vi "Write plots.vi"(5 "plots":refnum<class "Plot.lvclass">[](array[class]), 9 "WaveformChart in":refnum<class "WaveformChart.lvclass">) -> (3 "WaveformChart out":refnum<class "WaveformChart.lvclass">)   [LabVIEW 2014, in "WaveformChart.lvclass"]
uses:
  WaveformChart.lvclass
  Plot/Plot.lvclass
  WaveformChart.lvclass/WaveformChart.ctl
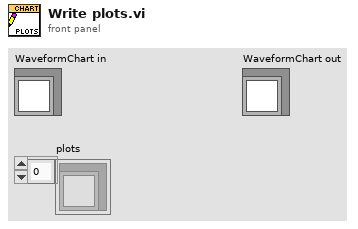
[diagram p1: front panel]
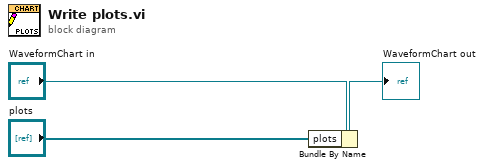
[diagram p0: block diagram]
diagram:
  n1 = Bundle By Name(cluster="WaveformChart in", "plots"="plots") -> (→"WaveformChart out":refnum<class "WaveformChart.lvclass">)
